vi "Impedance_Sweep_Freq.vi"() -> ()   [LabVIEW 2020]
uses:
  <vilib>/Math Plots/2D Math Plots/2D Compass/2D Compass XCtrl/2D Compass.xctl
  <vilib>/Analysis/1siggen.llb/Ramp Pattern by Samples.vi
  <vilib>/Analysis/baseanly.llb/Mean (DBL).vi
  <vilib>/Math Plots/2D Math Plots/2D Compass/2D Compass Datatype/Public/Plot Helper (Vector).vi
  <vilib>/Analysis/NI_AALBase.lvlib
  <vilib>/Math Plots/2D Math Plots/2D Compass/2D Compass Datatype/2D Compass Datatype.lvclass
panel:
  out "Progress":i32(slide) scale=0.0..100.0
  in  "Tab Control":enum32{"Inputs", "Outputs", "Additional Plots"}(tab)
  in  "Test Params Cluster":T1={"Test Freq. (Hz)"=0.0, "Output Signal Amplitude\nVolts Pk"=0.1, "Sampling Time (s)"=0.1, "Sampling Rate (Hz)"=2000000.0, "Output Channel"="PXI1Slot2/ao1", "Current Channel"="PXI1Slot2/ai1", "Voltage Channel"="PXI1Slot2/ai0", "Trigger Channel"="/PXI1Slot2/ao/StartTrigger", "Number of runs"=5} {"Output Signal Amplitude\nVolts Pk" format="%#_6p"; "Sampling Time (s)" format="%#_6p"; "Sampling Rate (Hz)" format="%#_6p"}
  in  "Stop Freq":dbl=50000.0 format="%#.4p"
  in  "Start Freq":dbl=100.0 format="%#.4p"
  in  "Number of\nTest Freqs":i32=128
  out "Test Number":i32=8
  in  "LCR Params":T2={"Rg_Vmon"=5000.0, "Rg_Imon"=5000.0, "ESL_Cal"=2.5e-07, "ESR_Cal"=0.0, "Cp_Cal"=0.0, "Rp_Cal"=1000000000.0, "UseCorrection"=TRUE, "R_Shunt"=100.0} {"R_Shunt" format="%#_6p"; "Rg_Vmon" format="%#_6p"; "Rg_Imon" format="%#_6p"; "ESL_Cal" format="%#_6p"; "ESR_Cal" format="%#_6p"; "Cp_Cal" format="%#_6p"; "Rp_Cal" format="%#_6p"}
  in  "Path":path=path "C:/Users/Human-MPI/Desktop/Temp"
  in  "File Name String":string="Test"
  in  "Experiment Title":string="Experiment Title"
  in  "Save Data?":bool
  in  "type":u16(ring)=1 items=["Linear", "Logarithmic"]
  out "Single Run \nImpedance Cluster":T3={"|Z|"=nan, "Phase(Z)"=nan, "Re(Z)"=nan, "Imag(Z)"=nan, "Ls"=nan, "Cs"=nan, "Rp"=0.0, "Cp"=0.0} {"|Z|" format="%#_5p"; "Phase(Z)" format="%#_5p"; "Re(Z)" format="%#_5p"; "Imag(Z)" format="%#_5p"; "Ls" format="%#_5p"; "Cs" format="%#_5p"; "Rp" format="%#_5p"; "Cp" format="%#_5p"}
  out "Mean Mag":dbl format="%.4p"
  out "Mean Phase":dbl format="%0.2f"
  out "Mag Phase Graph":cluster{dbl[], dbl[]}[](graph)
  out "RealImag Graph":cluster{dbl[], dbl[]}[](graph)
  out "2D Compass":refnum<class "2D Plot Datatype.lvclass">[](xcontrol)
  out "output cluster":T1={"Test Freq. (Hz)"=3243.3070866141734, "Output Signal Amplitude\nVolts Pk"=0.1, "Sampling Time (s)"=0.01, "Sampling Rate (Hz)"=250000.0, "Output Channel"="Dev3/ao0", "Current Channel"="Dev3/ai1", "Voltage Channel"="Dev3/ai0", "Trigger Channel"="/Dev3/ao/StartTrigger", "Number of runs"=5}
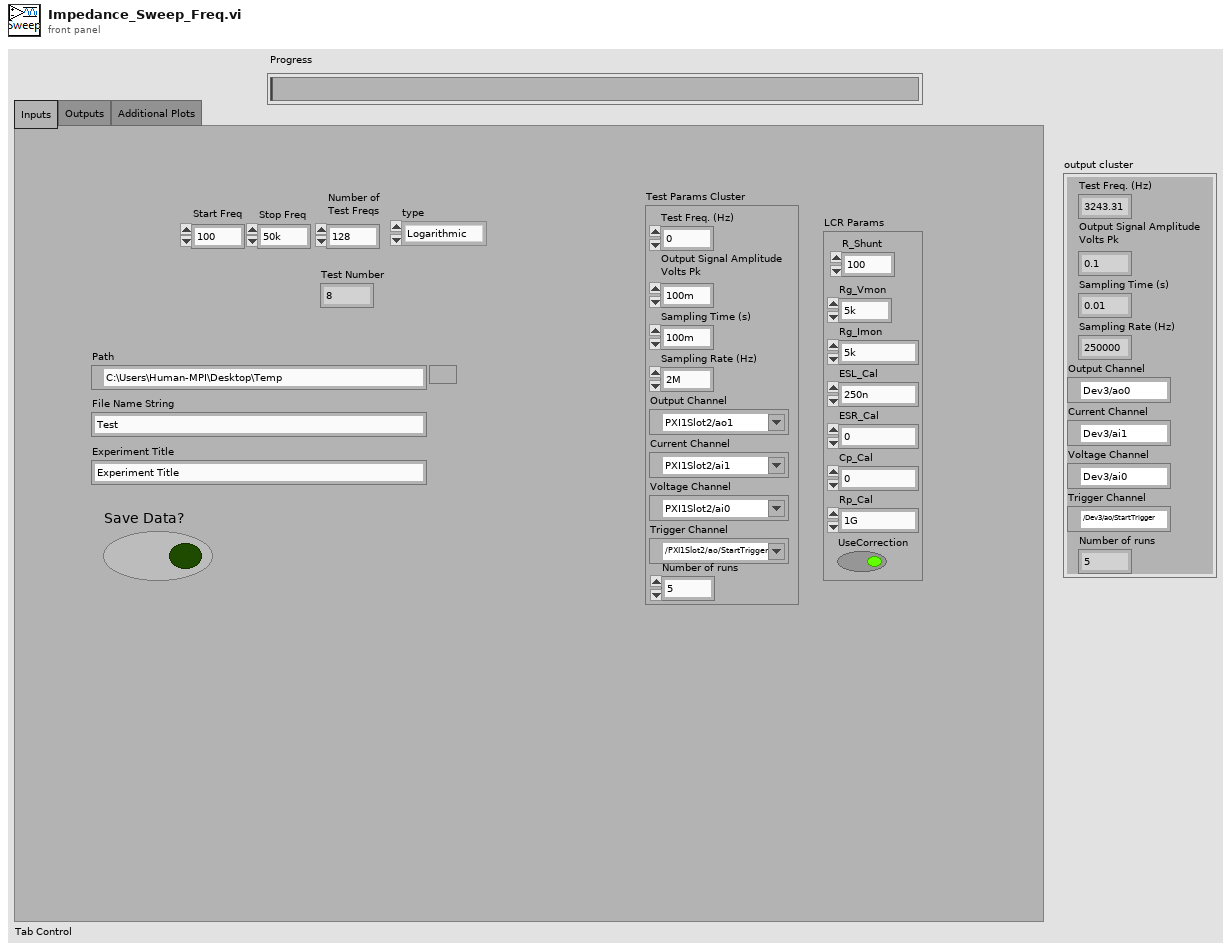
[diagram p1: front panel]
types:
  T1 = cluster{"Test Freq. (Hz)":dbl, "Output Signal Amplitude\nVolts Pk":dbl, "Sampling Time (s)":dbl, "Sampling Rate (Hz)":dbl, "Output Channel":tag, "Current Channel":tag, "Voltage Channel":tag, "Trigger Channel":tag, "Number of runs":i32}
  T2 = cluster{"Rg_Vmon":dbl, "Rg_Imon":dbl, "ESL_Cal":dbl, "ESR_Cal":dbl, "Cp_Cal":dbl, "Rp_Cal":dbl, "UseCorrection":bool, "R_Shunt":dbl}
  T3 = cluster{"|Z|":dbl, "Phase(Z)":dbl, "Re(Z)":dbl, "Imag(Z)":dbl, "Ls":dbl, "Cs":dbl, "Rp":dbl, "Cp":dbl}
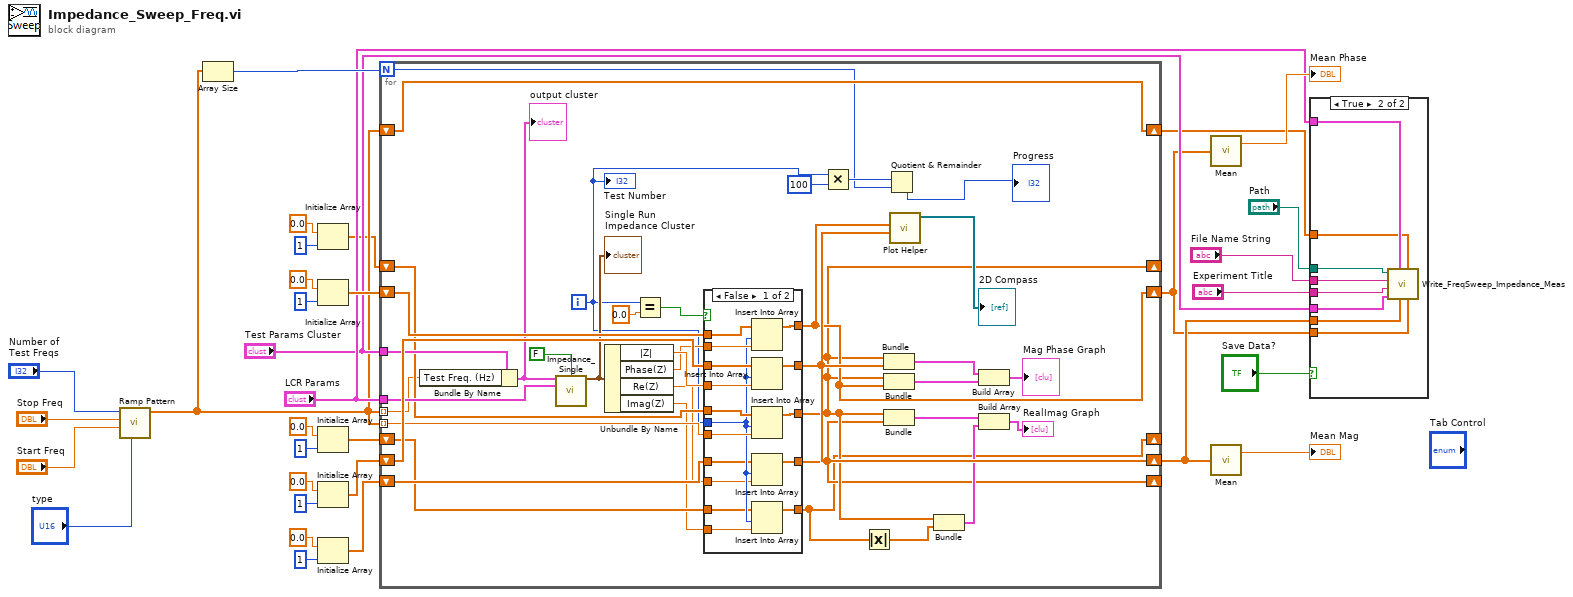
[diagram p0: block diagram]
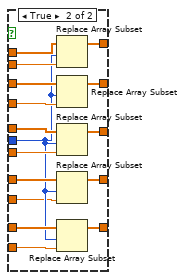
[diagram p3: hidden frame]
diagram:
  n1 = call-poly <vilib>:"Ramp Pattern.vi"("type"="type", "start"="Start Freq", "end"="Stop Freq", "samples"="Number of\nTest Freqs") -> ("Ramp Pattern"=w10:dbl[])  [unwired: 6 in, 1 out]
  n2 = Array Size(array=w10) -> (size(s)=w25:i32)
  n3 = Initialize Array(0.0 ("element"), 1 ("dimension size")) -> (w7:dbl[])
  n4 = Initialize Array(0.0 ("element"), 1 ("dimension size")) -> (w24:dbl[])
  n5 = Initialize Array(0.0 ("element"), 1 ("dimension size")) -> (w1:dbl[])
  n6 = Initialize Array(0.0 ("element"), 1 ("dimension size")) -> (w27:dbl[])
  n7 = Initialize Array(0.0 ("element"), 1 ("dimension size")) -> (w2:dbl[])
  n8 = for {
    N: w25 -> [w34]
    tunnel: w10 -> [w56] mode=indexing
    shift-right: [w51] -> w13
    shift-left: w27 -> [w69]
    shift-right: [w50] -> w12
    shift-left: w24 -> [w68]
    shift-right: [w58] -> w11
    shift-left: w10 -> [w58]
    tunnel: "Test Params Cluster" -> [w60]
    tunnel: "LCR Params" -> [w67]
    tunnel: w10 -> [w53] mode=indexing
    shift-right: [w41] -> _
    shift-left: w7 -> [w57]
    shift-right: [w38] -> _
    shift-left: w1 -> [w47]
    shift-right: [w40] -> _
    shift-left: w2 -> [w48]
    i -> [w33]
    n9 = Bundle By Name(cluster=w60, "Test Freq. (Hz)"=w53) -> (w59:T1)
    "output cluster" <- w59
    n10 = call "Impedance_Single.vi"("Test Params Cluster"=w59, "SaveFile?"=FALSE, "LCR Params"=w67) -> ("Mean Signal\nImpedance cluster"=w65:T3)  [unwired: 12 in]
    "Single Run \nImpedance Cluster" <- w65
    n11 = Unbundle By Name(w65) -> ("|Z|"=w64:dbl, "Phase(Z)"=w63:dbl, "Re(Z)"=w46:dbl, "Imag(Z)"=w45:dbl)
    n12 = Equal?(x=w33, y=0.0) -> (x = y?=w61:bool)
    n13 = case shown="False" w61 {
      tunnel: w69 -> [w84 w101]
      tunnel: w68 -> [w85 w100]
      tunnel: [w77 w99] -> w50
      tunnel: [w81 w98] -> w51
      tunnel: w64 -> [w83 w97]
      tunnel: w63 -> [w82 w96]
      tunnel: w33 -> [w76 w90]
      tunnel: w57 -> [w80 w94]
      tunnel: w56 -> [w79 w93]
      tunnel: [w78 w95] -> w41
      tunnel: w48 -> [w75 w92]
      tunnel: w47 -> [w74 w91]
      tunnel: w46 -> [w73 w88]
      tunnel: w45 -> [w72 w89]
      tunnel: [w71 w87] -> w40
      tunnel: [w70 w86] -> w38
      frame False {
        n14 = Insert Into Array(array=w85, index=w76, new element=w82) -> (w77:dbl[])
        n15 = Insert Into Array(array=w84, index=w76, new element=w83) -> (w81:dbl[])
        n16 = Insert Into Array(array=w80, index=w76, new element=w79) -> (w78:dbl[])
        n17 = Insert Into Array(array=w75, index=w76, new element=w73) -> (w71:dbl[])
        n18 = Insert Into Array(array=w74, index=w76, new element=w72) -> (w70:dbl[])
      }
      frame True {
        n19 = Replace Array Subset(array=w100, new element=w96, index=w90) -> (w99:dbl[])
        n20 = Replace Array Subset(array=w101, new element=w97, index=w90) -> (w98:dbl[])
        n21 = Replace Array Subset(array=w94, new element=w93, index=w90) -> (w95:dbl[])
        n22 = Replace Array Subset(array=w92, new element=w88, index=w90) -> (w87:dbl[])
        n23 = Replace Array Subset(array=w91, new element=w89, index=w90) -> (w86:dbl[])
      }
    }
    n24 = Multiply(x=w33, y=100) -> (x*y=w35:i32)
    n25 = Absolute Value(x=w38) -> (abs(x)=w39:dbl[])
    n26 = Bundle(w41, w51) -> (w49:cluster{dbl[], dbl[]})  [unwired: 1 in]
    n27 = Bundle(w41, w50) -> (w54:cluster{dbl[], dbl[]})  [unwired: 1 in]
    n28 = Bundle(w41, w40) -> (w44:cluster{dbl[], dbl[]})  [unwired: 1 in]
    n29 = Quotient & Remainder(x=w35, y=w34) -> (floor(x/y)=→"Progress":i32)  [unwired: 1 out]
    n30 = call-poly <vilib>:"Plot Helper.vi"("radius vector"=w51, "theta vector"=w50) -> ("2D Plot Class Obj Array out"=→"2D Compass":refnum<class "2D Plot Datatype.lvclass">[])  [unwired: 2 in, 7 out]
    n31 = Bundle(w41, w39) -> (w43:cluster{dbl[], dbl[]})  [unwired: 1 in]
    n32 = Build Array(w49, w54) -> (→"Mag Phase Graph":cluster{dbl[], dbl[]}[])
    n33 = Build Array(w44, w43) -> (→"RealImag Graph":cluster{dbl[], dbl[]}[])
    "Test Number" <- w33
  }
  n34 = call-poly <vilib>:"Mean.vi"("X"=w12) -> ("mean"=→"Mean Phase":dbl)  [unwired: 1 out]
  n35 = call-poly <vilib>:"Mean.vi"("X"=w13) -> ("mean"=→"Mean Mag":dbl)  [unwired: 1 out]
  n36 = case shown="True" "Save Data?" {
    tunnel: "LCR Params" -> [_ w109]
    tunnel: "Path" -> [_ w108]
    tunnel: "File Name String" -> [_ w107]
    tunnel: "Experiment Title" -> [_ w106]
    tunnel: "Test Params Cluster" -> [_ w105]
    tunnel: w13 -> [_ w103]
    tunnel: w12 -> [_ w102]
    tunnel: w11 -> [_ w104]
    frame False {
    }
    frame True {
      n37 = call "Write_FreqSweep_Impedance_Meas.vi"("Z_Phase_Vec"=w102, "Freq Vector"=w104, "|Z| Vector"=w103, "Compensation and Gain"=w109, "Test Params Cluster"=w105, "Experiment Title"=w106, "File Name String"=w107, "Path"=w108) -> ()  [unwired: 4 in]
    }
  }
